vi "Close.vi"(0 "VISA resource name":refnum<visa-resource-name>, 1 "Query For SCPI Errors? (T)":bool=TRUE, 11 "error in (no error)":errorcluster) -> (15 "error out":errorcluster)   [LabVIEW 2014, in "KE6514Driver.lvlib"]
doc: "Performs an instrument error query before terminating the software connection to the instrument."
uses:
  KE6514Driver.lvlib
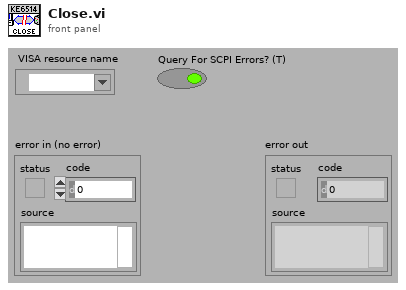
[diagram p1: front panel]
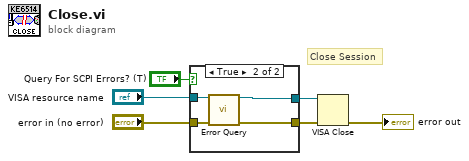
[diagram p0: block diagram]
diagram:
  # "Close Session"
  n1 = case shown="True" "Query For SCPI Errors? (T)" {
    tunnel: "VISA resource name" -> [w8 w12]
    tunnel: "error in (no error)" -> [w7 w11]
    tunnel: [w7 w10] -> w3
    tunnel: [w8 w9] -> w2
    frame False {
    }
    frame True {
      n2 = call "Error Query.vi"("VISA Resource In"=w12, "error in (no error)"=w11) -> ("VISA Resource Out (dupl)"=w9:refnum<visa-resource-name>, "error out"=w10:errorcluster)  [unwired: 10 in, 2 out]
    }
  }
  n3 = VISA Close(VISA resource name=w2, error in (no error)=w3) -> (error out=→"error out":errorcluster)
